vi "ProgramaPrincipal.vi"() -> ()   [LabVIEW 2018]
uses:
  Start Button.xctl
  <vilib>/Utility/file.llb/Write Delimited Spreadsheet (string).vi
panel:
  out "Boolean 2":bool=TRUE
  out "Boolean":bool=TRUE
  in  "Tab Control":enum32{"Modo usuario", "Modo administrador"}(tab)
  out "Temperatura °C":dbl
  out "Grafica de temperatura":dbl(graph)
  in  "Limite superior de Temperatura °C":dbl=100.0
  in  "Limite inferior de Temperatura °C":dbl
  out "Alarma":string
  out "Alarma HIG TEMPERATURE":string
  out "Alarma LOW TEMPERATURE":string
  in  "Start Button":dbl(xcontrol)
  in  "Temperatura °C":dbl=36.0
  out "Temperatura °F":dbl
  out "Temperatura aleatoria °C":dbl
  in  "Tiempo de muestreo del FILE/IO (ms)":u32=1000
  in  "checkbox adquiridos":bool
  in  "Tiempo de muestreo de la alarma (ms)":u32=1000
  in  "Checkbox alertas":bool
  in  "Tiempo de muestreo del sensor (ms)":u32=100
  out "Voltaje del sensor":dbl format="%f Voltios"
  in  "Modo MANUAL/AUTOMATICO":bool
  in  "STOP":bool
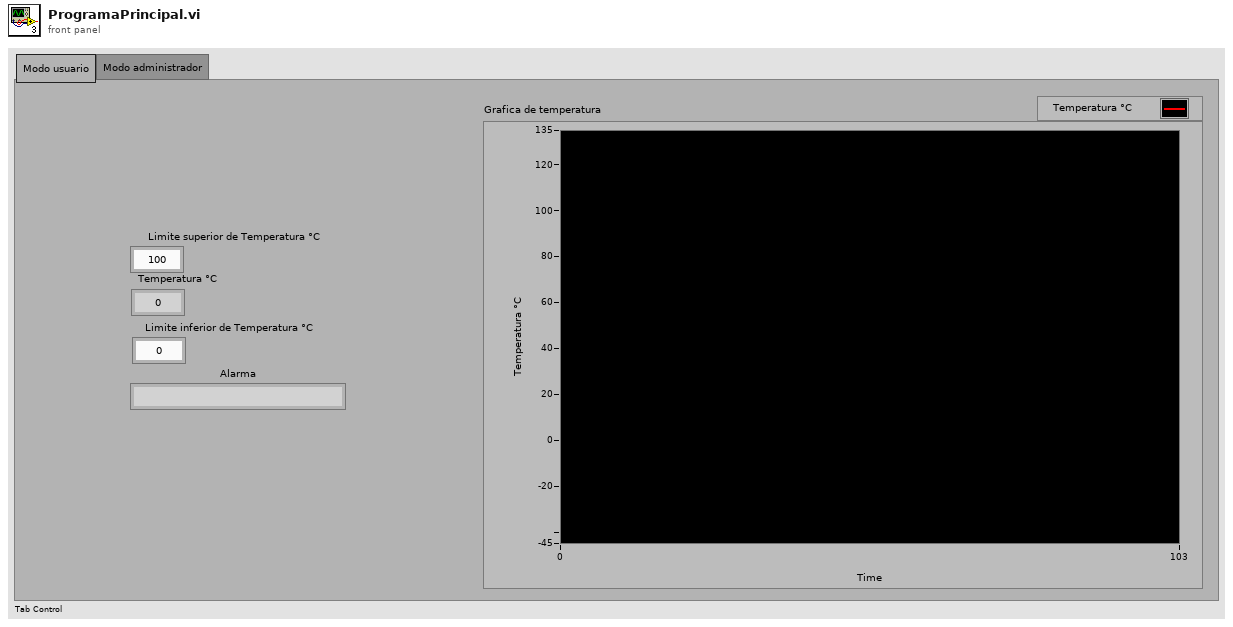
[diagram p1: front panel]
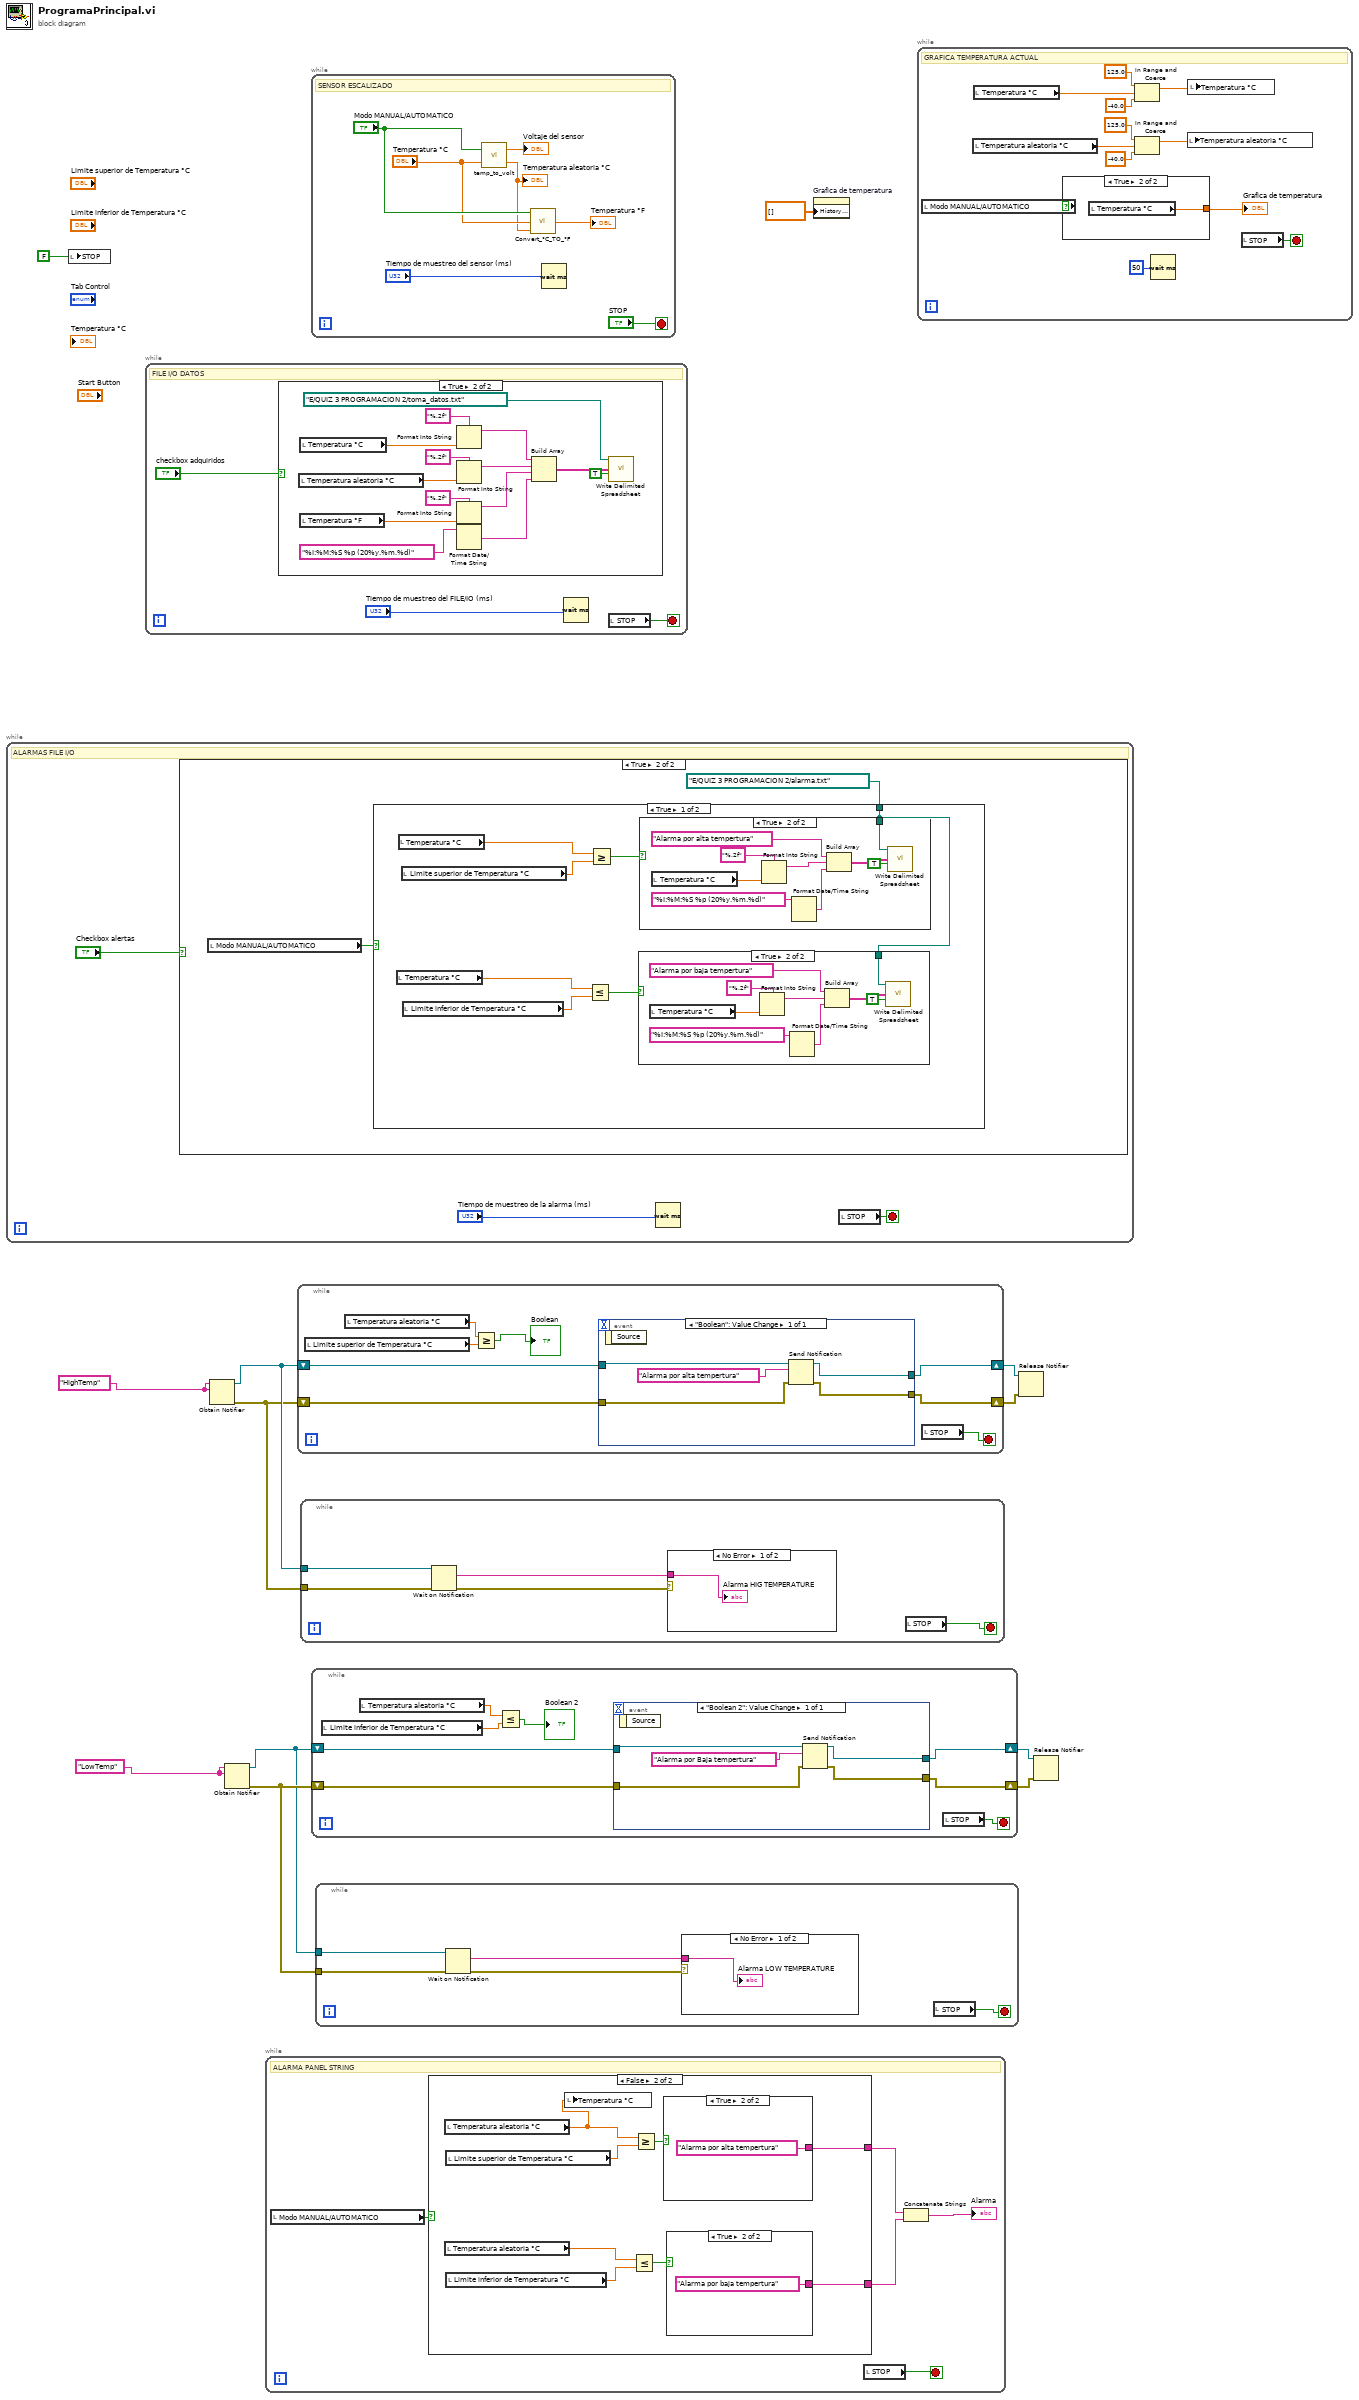
[diagram p0: block diagram]
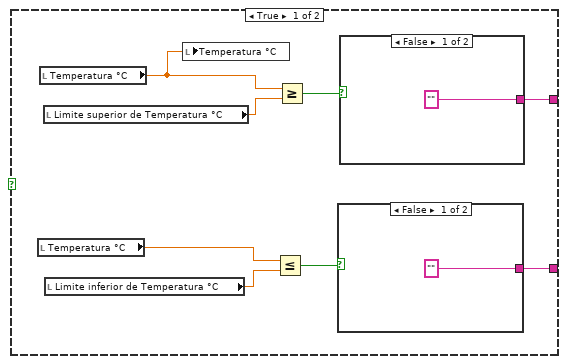
[diagram p4: hidden frame]
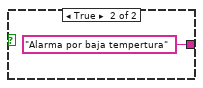
[diagram p5: hidden frame]
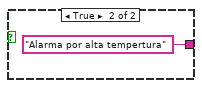
[diagram p6: hidden frame]
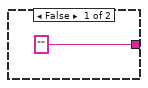
[diagram p7: hidden frame]
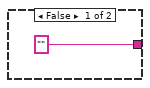
[diagram p8: hidden frame]
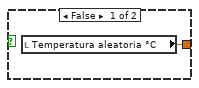
[diagram p9: hidden frame]
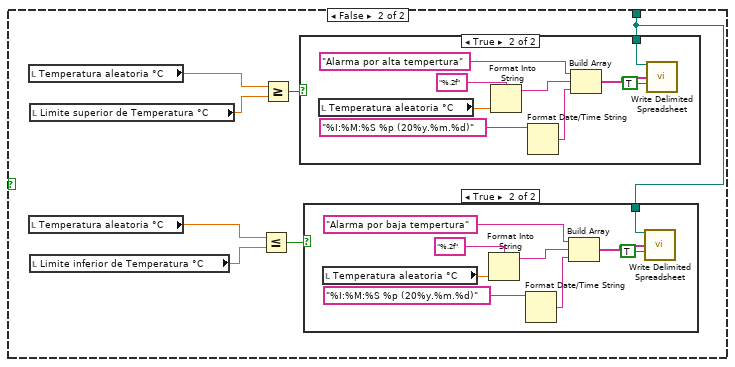
[diagram p13: hidden frame]
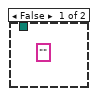
[diagram p15: hidden frame]
diagram:
  w5 = "LowTemp" ("name (unnamed)")
  w6 = "HighTemp" ("name (unnamed)")
  n1 = while {
    stop <- w13 stop-if-true
    # "ALARMAS FILE I/O"
    n2 = case shown="True" "Checkbox alertas" {
      frame False {
      }
      frame True {
        n3 = local read "Modo MANUAL/AUTOMATICO"() -> (w17:bool)
        n4 = case shown="True" w17 {
          tunnel: path "E:/QUIZ 3 PROGRAMACION 2/alarma.txt" ("file path (dialog if empty)") -> [w18 w43]
          frame True {
            n5 = local read "Temperatura °C"() -> (w19:dbl)
            n6 = local read "Temperatura °C"() -> (w24:dbl)
            n7 = local read "Limite superior de Temperatura °C"() -> (w22:dbl)
            n8 = local read "Limite inferior de Temperatura °C"() -> (w21:dbl)
            n9 = Less Or Equal?(x=w19, y=w21) -> (x <= y?=w20:bool)
            n10 = Greater Or Equal?(x=w24, y=w22) -> (x >= y?=w23:bool)
            n11 = case shown="True" w20 {
              tunnel: w18 -> [_ w27]
              frame False {
              }
              frame True {
                n12 = local read "Temperatura °C"() -> (w29:dbl)
                n13 = Format Into String(format string="%.2f", w29) -> (resulting string=w28:string)  [unwired: 2 in, 1 out]
                n14 = Format Date/Time String(time format string (%c)="%I:%M:%S %p (20%y.%m.%d)") -> (date/time string=w30:string)  [unwired: 2 in]
                n15 = Build Array("Alarma por baja tempertura", w28, w30) -> (w32:string[])
                n16 = call-poly <vilib>:"Write Delimited Spreadsheet.vi"("file path (dialog if empty)"=w27, "1D data"=w32, "append to file? (new file:F)"=TRUE) -> ()  [unwired: 11 in, 2 out]
              }
            }
            n17 = case shown="True" w23 {
              tunnel: w18 -> [_ w39]
              frame False {
              }
              frame True {
                n18 = local read "Temperatura °C"() -> (w37:dbl)
                n19 = Format Into String(format string="%.2f", w37) -> (resulting string=w36:string)  [unwired: 2 in, 1 out]
                n20 = Format Date/Time String(time format string (%c)="%I:%M:%S %p (20%y.%m.%d)") -> (date/time string=w38:string)  [unwired: 2 in]
                n21 = Build Array("Alarma por alta tempertura", w36, w38) -> (w41:string[])
                n22 = call-poly <vilib>:"Write Delimited Spreadsheet.vi"("file path (dialog if empty)"=w39, "1D data"=w41, "append to file? (new file:F)"=TRUE) -> ()  [unwired: 11 in, 2 out]
              }
            }
          }
          frame False {
            n23 = local read "Temperatura aleatoria °C"() -> (w49:dbl)
            n24 = local read "Temperatura aleatoria °C"() -> (w44:dbl)
            n25 = local read "Limite superior de Temperatura °C"() -> (w47:dbl)
            n26 = local read "Limite inferior de Temperatura °C"() -> (w46:dbl)
            n27 = Less Or Equal?(x=w44, y=w46) -> (x <= y?=w45:bool)
            n28 = Greater Or Equal?(x=w49, y=w47) -> (x >= y?=w48:bool)
            n29 = case shown="True" w48 {
              tunnel: w43 -> [_ w64]
              frame False {
                (unwired) ""
              }
              frame True {
                n30 = local read "Temperatura aleatoria °C"() -> (w62:dbl)
                n31 = Format Into String(format string="%.2f", w62) -> (resulting string=w61:string)  [unwired: 2 in, 1 out]
                n32 = Format Date/Time String(time format string (%c)="%I:%M:%S %p (20%y.%m.%d)") -> (date/time string=w63:string)  [unwired: 2 in]
                n33 = Build Array "Build Array"("Alarma por alta tempertura", w61, w63) -> (w66:string[])
                n34 = call-poly <vilib>:"Write Delimited Spreadsheet.vi"("file path (dialog if empty)"=w64, "1D data"=w66, "append to file? (new file:F)"=TRUE) -> ()  [unwired: 11 in, 2 out]
              }
            }
            n35 = case shown="True" w45 {
              tunnel: w43 -> [_ w52]
              frame False {
              }
              frame True {
                n36 = local read "Temperatura aleatoria °C"() -> (w54:dbl)
                n37 = Format Into String(format string="%.2f", w54) -> (resulting string=w53:string)  [unwired: 2 in, 1 out]
                n38 = Format Date/Time String(time format string (%c)="%I:%M:%S %p (20%y.%m.%d)") -> (date/time string=w55:string)  [unwired: 2 in]
                n39 = Build Array("Alarma por baja tempertura", w53, w55) -> (w57:string[])
                n40 = call-poly <vilib>:"Write Delimited Spreadsheet.vi"("file path (dialog if empty)"=w52, "1D data"=w57, "append to file? (new file:F)"=TRUE) -> ()  [unwired: 11 in, 2 out]
              }
            }
          }
        }
      }
    }
    n41 = Wait (ms)(milliseconds to wait="Tiempo de muestreo de la alarma (ms)") -> ()  [unwired: 1 out]
    n42 = local read "STOP"() -> (w13:bool)
  }
  n43 = local write "STOP"(FALSE) -> ()
  n44 = while {
    stop <- w68 stop-if-true
    # "FILE I/O DATOS"
    n45 = case shown="True" "checkbox adquiridos" {
      frame False {
      }
      frame True {
        n46 = local read "Temperatura aleatoria °C"() -> (w82:dbl)
        n47 = local read "Temperatura °C"() -> (w83:dbl)
        n48 = local read "Temperatura °F"() -> (w81:dbl)
        n49 = Format Into String(format string="%.2f", w83) -> (resulting string=w80:string)  [unwired: 2 in, 1 out]
        n50 = Format Into String(format string="%.2f", w82) -> (resulting string=w78:string)  [unwired: 2 in, 1 out]
        n51 = Format Into String(format string="%.2f", w81) -> (resulting string=w77:string)  [unwired: 2 in, 1 out]
        n52 = Format Date/Time String(time format string (%c)="%I:%M:%S %p (20%y.%m.%d)") -> (date/time string=w79:string)  [unwired: 2 in]
        n53 = Build Array(w80, w78, w77, w79) -> (w76:string[])
        n54 = call-poly <vilib>:"Write Delimited Spreadsheet.vi"("file path (dialog if empty)"=path "E:/QUIZ 3 PROGRAMACION 2/toma_datos.txt", "1D data"=w76, "append to file? (new file:F)"=TRUE) -> ()  [unwired: 11 in, 2 out]
      }
    }
    n55 = Wait (ms)(milliseconds to wait="Tiempo de muestreo del FILE/IO (ms)") -> ()  [unwired: 1 out]
    n56 = local read "STOP"() -> (w68:bool)
  }
  n57 = Obtain Notifier(name (unnamed)=w6, notification data type=w6) -> (notifier out=w8:refnum<notifier>, error out=w7:errorcluster)  [unwired: 2 in, 1 out]
  n58 = Obtain Notifier(name (unnamed)=w5, notification data type=w5) -> (notifier out=w3:refnum<notifier>, error out=w4:errorcluster)  [unwired: 2 in, 1 out]
  n59 = while {
    stop <- w85 stop-if-true
    # "ALARMA PANEL STRING"
    n60 = local read "Modo MANUAL/AUTOMATICO"() -> (w89:bool)
    n61 = case shown="False" w89 {
      tunnel: [w92 w104] -> w87
      tunnel: [w91 w103] -> w86
      frame True {
        n62 = local read "Temperatura °C"() -> (w93:dbl)
        n63 = local read "Temperatura °C"() -> (w90:dbl)
        n64 = local read "Limite superior de Temperatura °C"() -> (w96:dbl)
        n65 = local read "Limite inferior de Temperatura °C"() -> (w95:dbl)
        n66 = local write "Temperatura °C"(w90) -> ()
        n67 = Less Or Equal?(x=w93, y=w95) -> (x <= y?=w94:bool)
        n68 = Greater Or Equal?(x=w90, y=w96) -> (x >= y?=w97:bool)
        n69 = case shown="False" w94 {
          tunnel: ["" "Alarma por baja tempertura"] -> w91
          frame False {
          }
          frame True {
          }
        }
        n70 = case shown="False" w97 {
          tunnel: ["" "Alarma por alta tempertura"] -> w92
          frame False {
          }
          frame True {
          }
        }
      }
      frame False {
        n71 = local read "Temperatura aleatoria °C"() -> (w102:dbl)
        n72 = local read "Temperatura aleatoria °C"() -> (w105:dbl)
        n73 = local read "Limite superior de Temperatura °C"() -> (w108:dbl)
        n74 = local read "Limite inferior de Temperatura °C"() -> (w107:dbl)
        n75 = local write "Temperatura °C"(w102) -> ()
        n76 = Less Or Equal?(x=w105, y=w107) -> (x <= y?=w106:bool)
        n77 = Greater Or Equal?(x=w102, y=w108) -> (x >= y?=w109:bool)
        n78 = case shown="True" w109 {
          tunnel: ["" "Alarma por alta tempertura"] -> w104
          frame False {
          }
          frame True {
          }
        }
        n79 = case shown="True" w106 {
          tunnel: ["" "Alarma por baja tempertura"] -> w103
          frame False {
          }
          frame True {
          }
        }
      }
    }
    n80 = local read "STOP"() -> (w85:bool)
    n81 = Concatenate Strings "Concatenate Strings"(w87, w86) -> (→"Alarma":string)
  }
  n82 = while {
    shift-right: [w116] -> w9
    shift-left: w7 -> [w118]
    shift-right: [w117] -> w10
    shift-left: w8 -> [w119]
    stop <- w114 stop-if-true
    n83 = local read "Limite superior de Temperatura °C"() -> (w120:dbl)
    n84 = local read "Temperatura aleatoria °C"() -> (w121:dbl)
    n85 = Greater Or Equal?(x=w121, y=w120) -> (x >= y?=→"Boolean":bool)
    n86 = event shown="[0] \"Boolean\": Value Change" {
      selector: _ -> [_]
      dyn-events: _ -> [_]
      timeout: _ -> [_]
      tunnel: w119 -> [w125]
      tunnel: w118 -> [w124]
      tunnel: [w123] -> w117
      tunnel: [w122] -> w116
      event "Boolean": Value Change {
        n87 = event-data() -> ()  [unwired: 1 in, 1 out]
        n88 = Send Notification(notification="Alarma por alta tempertura", notifier=w125, error in (no error)=w124) -> (notifier out=w123:refnum<notifier>, error out=w122:errorcluster)
      }
    }
    n89 = local read "STOP"() -> (w114:bool)
  }
  n90 = while {
    tunnel: w8 -> [w131]
    tunnel: w7 -> [w130]
    stop <- w127 stop-if-true
    n91 = Wait on Notification(notifier=w131, error in (no error)=w130) -> (notification=w128:string, error out=w129:errorcluster)  [unwired: 2 in, 2 out]
    n92 = case shown="No Error" w129 {
      tunnel: w128 -> [w132 _]
      frame No Error {
        "Alarma HIG TEMPERATURE" <- w132
      }
      frame Error {
      }
    }
    n93 = local read "STOP"() -> (w127:bool)
  }
  n94 = while {
    stop <- "STOP" stop-if-true
    # "SENSOR ESCALIZADO"
    n95 = call "temp_to_volt.vi"("Temperatura °C"="Temperatura °C", "Manual/Automatico"="Modo MANUAL/AUTOMATICO") -> ("Temperatura aleatoria °c"=w134:dbl, "Voltaje"=→"Voltaje del sensor":dbl)
    "Temperatura aleatoria °C" <- w134
    n96 = call "Convert_°C_TO_°F.vi"("Temperatura aleatoria °c"=w134, "Temperatura °C"="Temperatura °C", "Manual/Automatico"="Modo MANUAL/AUTOMATICO") -> ("Temperatura °F"=→"Temperatura °F":dbl)
    n97 = Wait (ms)(milliseconds to wait="Tiempo de muestreo del sensor (ms)") -> ()  [unwired: 1 out]
  }
  n98 = while {
    shift-right: [w144] -> w2
    shift-left: w4 -> [w146]
    shift-right: [w145] -> w1
    shift-left: w3 -> [w147]
    stop <- w140 stop-if-true
    n99 = local read "Limite inferior de Temperatura °C"() -> (w142:dbl)
    n100 = local read "Temperatura aleatoria °C"() -> (w143:dbl)
    n101 = Less Or Equal?(x=w143, y=w142) -> (x <= y?=→"Boolean 2":bool)
    n102 = event shown="[0] \"Boolean 2\": Value Change" {
      selector: _ -> [_]
      dyn-events: _ -> [_]
      timeout: _ -> [_]
      tunnel: w147 -> [w151]
      tunnel: w146 -> [w150]
      tunnel: [w149] -> w145
      tunnel: [w148] -> w144
      event "Boolean 2": Value Change {
        n103 = event-data() -> ()  [unwired: 1 in, 1 out]
        n104 = Send Notification(notification="Alarma por Baja tempertura", notifier=w151, error in (no error)=w150) -> (notifier out=w149:refnum<notifier>, error out=w148:errorcluster)
      }
    }
    n105 = local read "STOP"() -> (w140:bool)
  }
  n106 = while {
    tunnel: w3 -> [w157]
    tunnel: w4 -> [w156]
    stop <- w153 stop-if-true
    n107 = Wait on Notification(notifier=w157, error in (no error)=w156) -> (notification=w154:string, error out=w155:errorcluster)  [unwired: 2 in, 2 out]
    n108 = case shown="No Error" w155 {
      tunnel: w154 -> [w158 _]
      frame No Error {
        "Alarma LOW TEMPERATURE" <- w158
      }
      frame Error {
      }
    }
    n109 = local read "STOP"() -> (w153:bool)
  }
  n110 = property on="Grafica de temperatura" class="WFChart (strict)"("History Data"=dbl[] []) -> ()  [unwired: 2 in, 2 out]
  n111 = while {
    stop <- w170 stop-if-true
    # "GRAFICA TEMPERATURA ACTUAL"
    n112 = local read "Modo MANUAL/AUTOMATICO"() -> (w169:bool)
    n113 = local read "Temperatura aleatoria °C"() -> (w162:dbl)
    n114 = local read "Temperatura °C"() -> (w165:dbl)
    n115 = case shown="True" w169 {
      tunnel: [w171 w172] -> w168
      frame False {
        n116 = local read "Temperatura aleatoria °C"() -> (w171:dbl)
      }
      frame True {
        n117 = local read "Temperatura °C"() -> (w172:dbl)
      }
    }
    "Grafica de temperatura" <- w168
    n118 = In Range and Coerce(upper limit=125.0, x=w165, lower limit=-40.0) -> (coerced(x)=w164:dbl)  [unwired: 1 out]
    n119 = In Range and Coerce(upper limit=125.0, x=w162, lower limit=-40.0) -> (coerced(x)=w163:dbl)  [unwired: 1 out]
    n120 = Wait (ms)(milliseconds to wait=u32 50) -> ()  [unwired: 1 out]
    n121 = local write "Temperatura aleatoria °C"(w163) -> ()
    n122 = local write "Temperatura °C"(w164) -> ()
    n123 = local read "STOP"() -> (w170:bool)
  }
  n124 = Release Notifier(notifier=w10, error in (no error)=w9) -> ()  [unwired: 1 in, 3 out]
  n125 = Release Notifier(notifier=w1, error in (no error)=w2) -> ()  [unwired: 1 in, 3 out]
